vi "Write Analogue.vi"(8 "error in (no error)":errorcluster, 10 "Output":bool, 11 "Keysight 5700C in":refnum<class "Keysight 5700C.lvclass">) -> (0 "error out":errorcluster, 3 "Keysight 5700C out":refnum<class "Keysight 5700C.lvclass">)   [LabVIEW 2019, in "Concrete.lvlib" / "Keysight 5700C.lvclass"]
uses:
  Keysight 5700C.lvclass
  Keysight 5700C.lvclass/Keysight 5700C.ctl
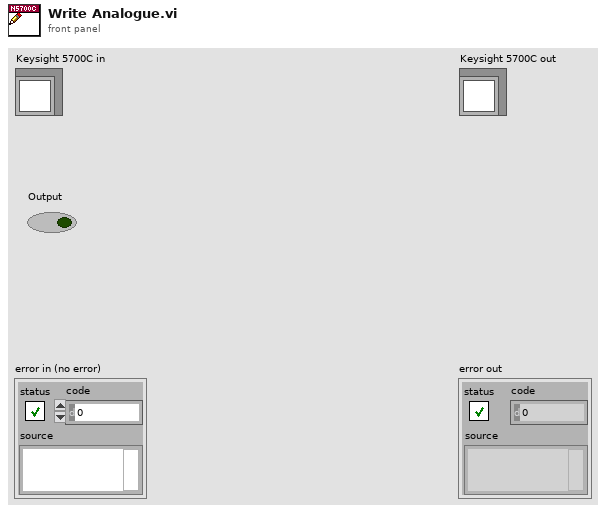
[diagram p1: front panel]
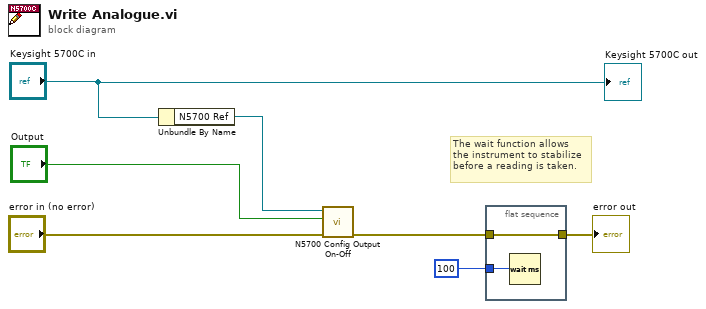
[diagram p0: block diagram]
diagram:
  # "The wait function allows \nthe instrument to stabilize\nbefore a reading is taken."
  n1 = Unbundle By Name("Keysight 5700C in") -> ("N5700 Ref"=w2:refnum<visa-resource-name>)
  n2 = call <instrlib>:"N5700 Config Output On-Off.vi"("error"="error in (no error)", "Output ON"="Output", "VISA"=w2) -> ("error out"=w1:errorcluster)  [unwired: 4 in, 1 out]
  n3 = flat-sequence {
    tunnel: [w9] -> w5
    tunnel: w1 -> [w9]
    tunnel: u32 100 ("milliseconds to wait") -> [w8]
    frame #0 {
      n4 = Wait (ms)(milliseconds to wait=w8) -> ()  [unwired: 1 out]
    }
  }
  "error out" <- w5
  "Keysight 5700C out" <- "Keysight 5700C in"
